vi "GenericMotionCore.vi"(5 "NumOfAxis":i32=3, 6 "MotorDisabled":refnum<vi>, 7 "Simulation":bool, 8 "error in":errorcluster, 9 "Serial Configuration":T1={"Baud Rate"=115200, "Parity"=0, "Data Bits"=8, "Stop Bits"=10, "Flow Control"=0} {"Flow Control" items=["None", "XON/XOFF", "RTS/CTS", "XON/XOFF & RTS/CTS", "DTR/DSR", "XON/XOFF & DTR/DSR"]; "Stop Bits" items=["1.0"=10, "1.5"=15, "2.0"=20]; "Data Bits" items=["7"=7, "8"=8]; "Parity" items=["None", "Odd", "Even", "Mark", "Space"]; "Baud Rate" items=["300"=300, "600"=600, "1200"=1200, "2400"=2400, "4800"=4800, "9600"=9600, "19200"=19200]}, 10 "CommPort":refnum<visa-resource-name>, 11 "ControlQueue in":refnum<queue>) -> (0 "error out":errorcluster, 3 "queue out":refnum<queue>)   [LabVIEW 2013, in "GenericMotionCore.lvlib"]
uses:
  <instrlib>/GenericMotionCore/GenericMotionCore.lvlib
  <instrlib>/GenericMotionCore/Public/Data/GenericMotion_State.ctl
  <instrlib>/GenericMotionCore/Public/Data/GenericMotion_Data.ctl
  <vilib>/Utility/error.llb/DialogType.ctl
  <instrlib>/GenericMotionCore/Public/Position_Generic.vi
panel:
  out "update_counter":i32
  in  "SoftReset":bool caption="Go"
  in  "Go_MoveRel":bool caption="Go"
  out "WaitStopBlink":i32
  out "tick_start":u32
  out "tick_stop":u32
  out "Returned_String":string
  out "refresh rate":i32
  in  "MotorDisabled":bool caption="Go"
  in  "Home":bool caption="Go"
  in  "StepWidth":dbl(ring)=0.2 items=["0.2 um"=0.0002, "0.001 mm"=0.001, "0.002 mm"=0.002, "0.005 mm "=0.005, "0.01 mm"=0.01, "0.02 mm"=0.02, "0.05 mm"=0.05, "0.1 mm"=0.1, "0.2 mm"=0.2, "1 mm"=1.0]
  in  "Z-":bool
  in  "Z+":bool
  in  "X+":bool
  in  "X-":bool
  in  "Y-":bool
  in  "Y+":bool
  in  "ClearErr":bool caption="Go"
  in  "STOP":bool caption="Go"
  in  "Quit":bool caption="Go"
  in  "SetPosition":dbl[](array[numeric])=[1.0, 1.0, 1.0] caption="Position" format="%.4f"
  in  "SetVelocity":dbl[](array[numeric])=[1.0] caption="Velocity"
  in  "SetAcceleration":dbl[](array[numeric])=[50.0] caption="Acceleration"
  in  "Go":bool
  out "Moving":bool
  out "Acceleration":dbl[](array[numeric])
  out "Velocity":dbl[](array[numeric])
  out "Position":dbl[](array[numeric])
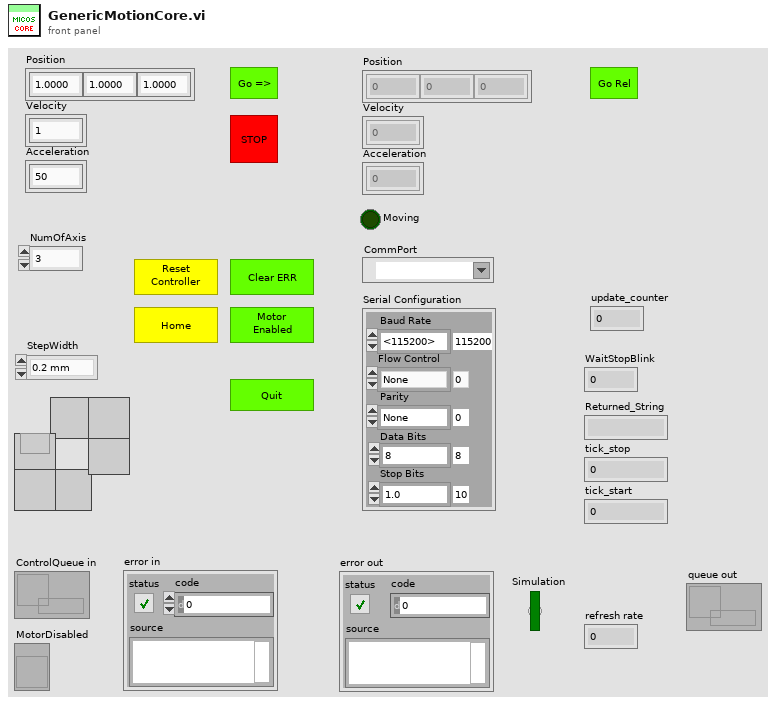
[diagram p1: front panel]
types:
  T1 = cluster{"Baud Rate":u32, "Parity":u16, "Data Bits":u16, "Stop Bits":u16, "Flow Control":u16}
  T2 = cluster{"Acceleration":dbl[], "Velocity":dbl[], "tick_move_target":u32, "Position target":dbl[], "Velocity_axial":dbl[]}
  T3 = cluster{"Position_Target":dbl[], "Velocity_axial":dbl[], "Acceleration":dbl[], "Moving":bool, "Simulation":bool, "tick_MoveTarget":u32, "NumOfAxis":i32, "Range":dbl[][]}
  T4 = cluster{"CommPort":refnum<vi>, "Serial Configuration":refnum<vi>, "SetPosition":refnum<vi>, "SetAcceleration":refnum<vi>, "SetVelocity":refnum<vi>, "StepWidth":refnum<vi>, "WaitStopReturn_Queue":refnum<queue>}
  T5 = typedef "GenericMotionCore.lvlib/GenericMotion_State.ctl" = cluster{"State":enum16{"Initialize", "SetDefaultConfig", "Close", "Quit", "Identify", "MoveAbs", "MoveAbs_all", "MoveRel", "MoveRel_all", "STOP", "Origin/Home", "WaitStop", "QueryStatus", "UpdateXPos", "UpdateAll", "SetVelocity", "SetAcceleration", "ClearErr", "LogMessage", "MotorEnable(1)", "EnableAxis", "JoyStick", "GetVelocity", "GetAcceleration", "SendCmd", "SetSoftLimits", "Beep", "_SettingReturn", "SoftReset"}, "Params.":variant}
  T6 = typedef "GenericMotionCore.lvlib/GenericMotion_Data.ctl" = cluster{"Position":dbl[], "Velocity":dbl[], "Acceleration":dbl[], "Moving":bool, "Simulation":bool, "tickcount_mov":u32, "tickcount_pos":u32, "NumOfAxis":i32, "Initialized":bool, "CommPort":refnum<visa-resource-name>, "Range":dbl[][], "Serial Configuration":cluster{"Baud Rate":u32, "Parity":u16, "Data Bits":u16, "Stop Bits":u16, "Flow Control":u16}, "MotorDisabled":refnum<vi>}
  T7 = typedef "StepWidthSelector.ctl" = dbl
  T8 = enum16{"Initialize", "SetDefaultConfig", "Close", "Quit", "Identify", "MoveAbs", "MoveAbs_all", "MoveRel", "MoveRel_all", "STOP", "Origin/Home", "WaitStop", "QueryStatus", "UpdateXPos", "UpdateAll", "SetVelocity", "SetAcceleration", "ClearErr", "LogMessage", "MotorEnable(1)", "EnableAxis", "JoyStick", "GetVelocity", "GetAcceleration", "SendCmd", "SetSoftLimits", "Beep", "_SettingReturn"}
  T9 = enum16{"Initialize", "SetDefaultConfig", "Close", "Quit", "Identify", "MoveAbs", "MoveAbs_all", "MoveRel", "MoveRel_all", "STOP", "Origin/Home", "WaitStop", "QueryStatus", "UpdateXPos", "UpdateAll", "SetVelocity", "SetAcceleration", "ClearErr", "LogMessage", "MotorEnable(1)", "EnableAxis", "JoyStick", "GetVelocity", "GetAcceleration", "SendCmd", "SetSoftLimits", "Beep", "_SettingReturn", "SoftReset"}
  T10 = typedef "DialogType.ctl" = u16
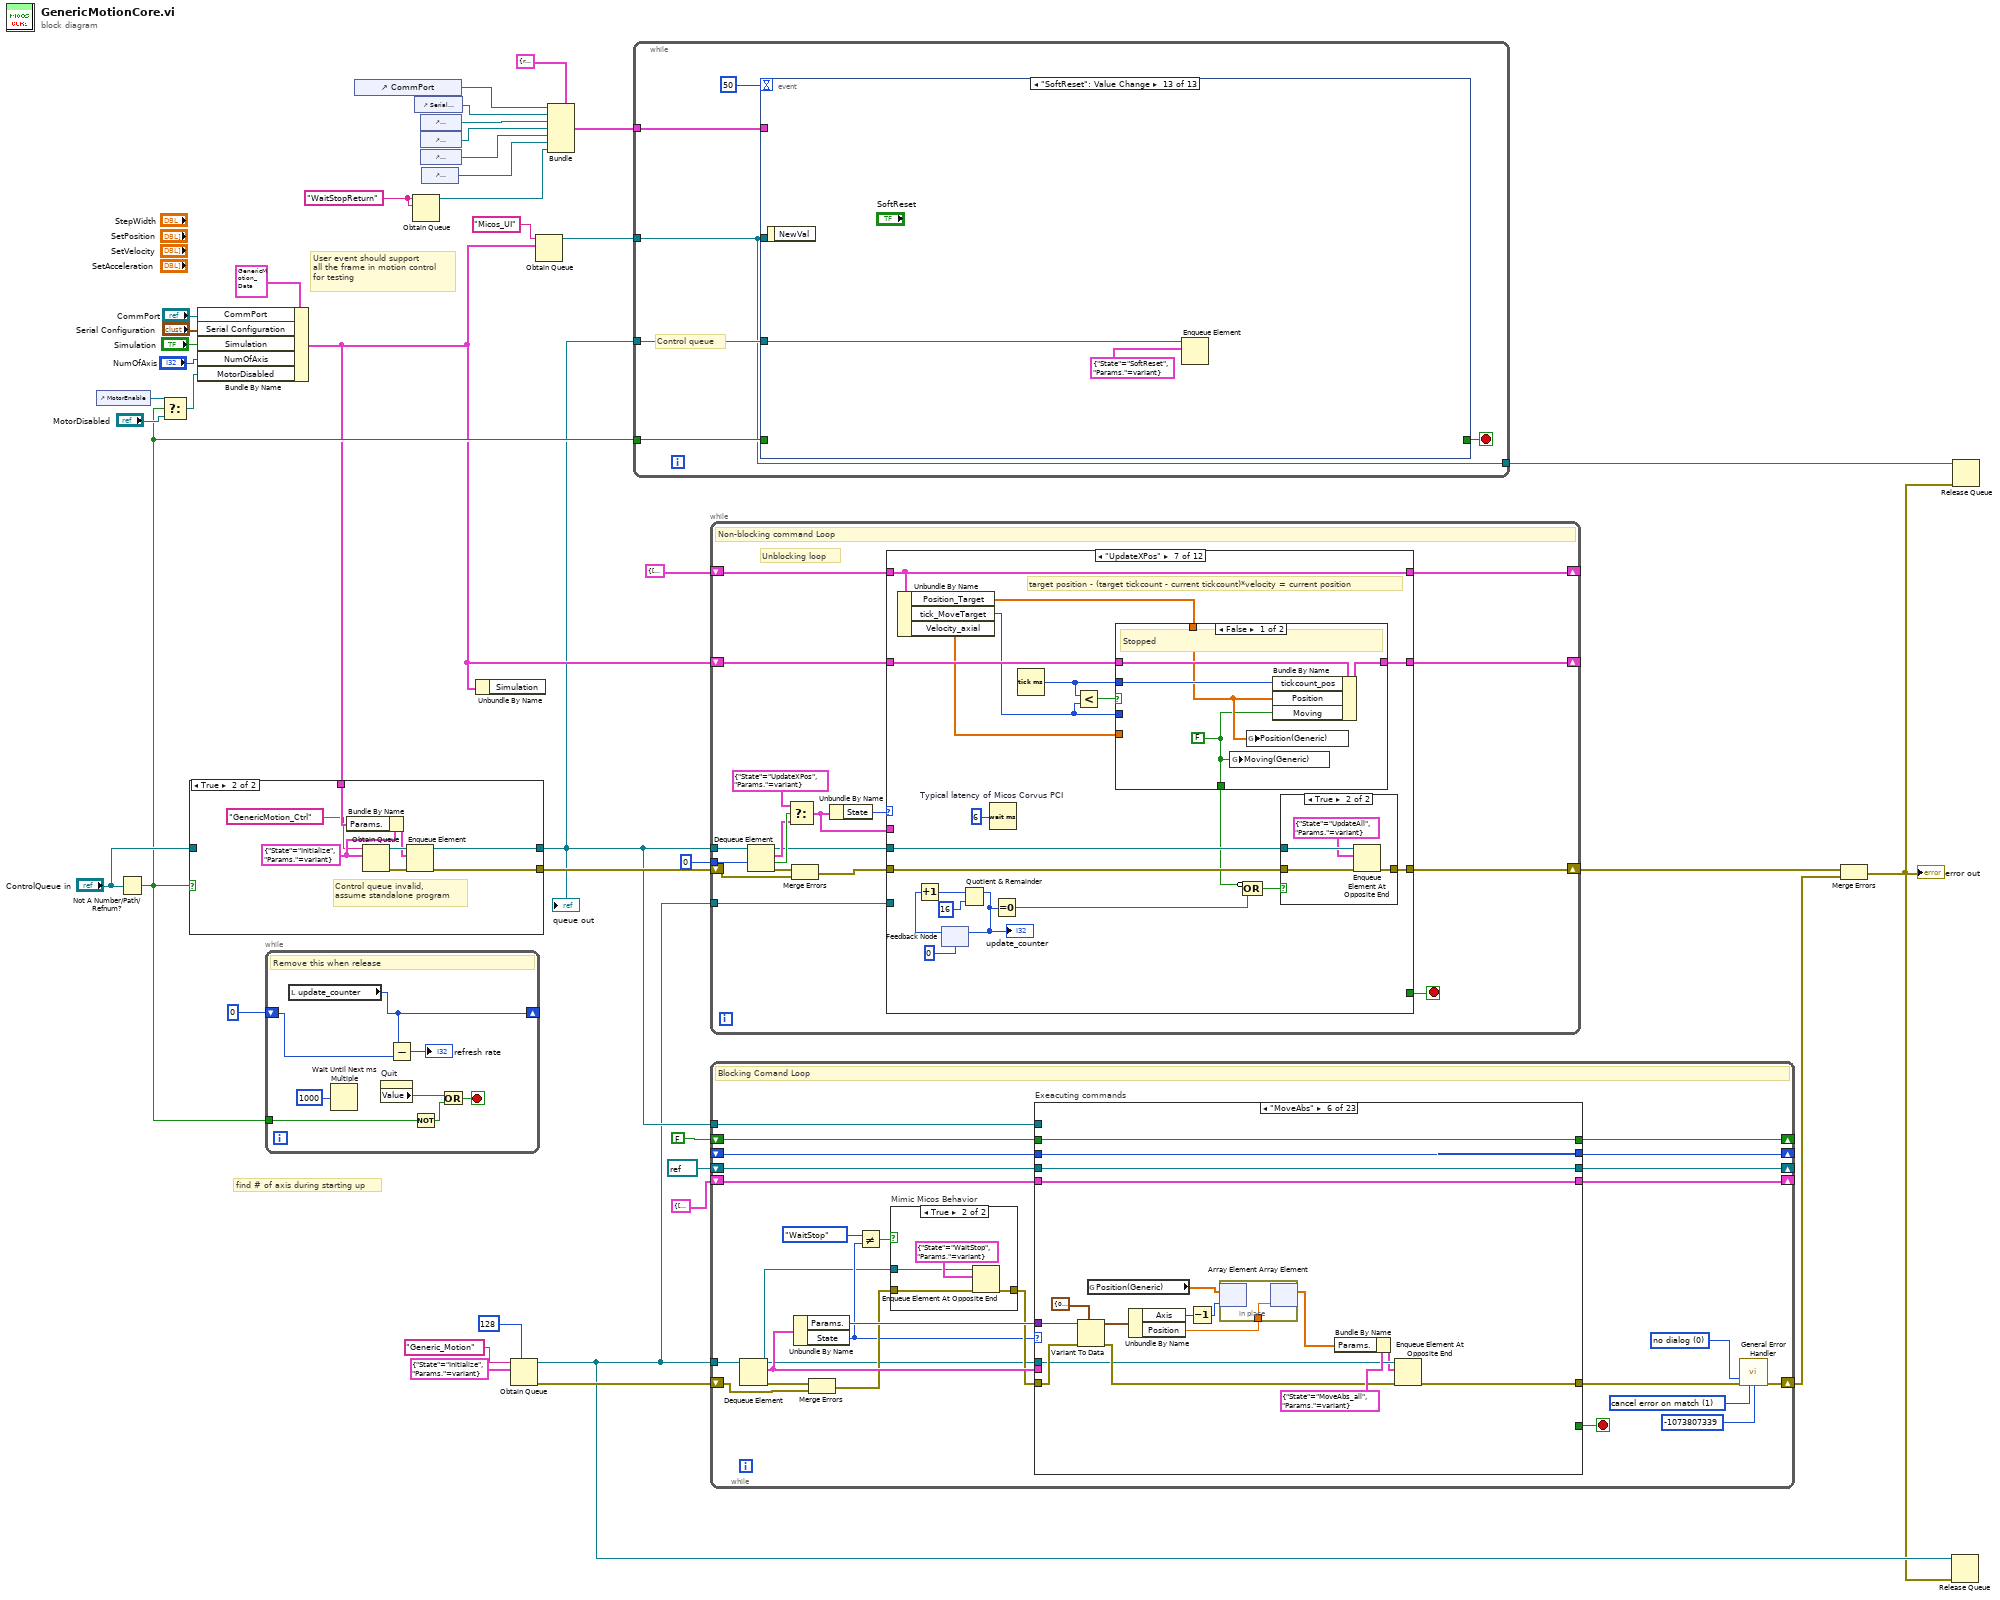
[diagram p0: block diagram]
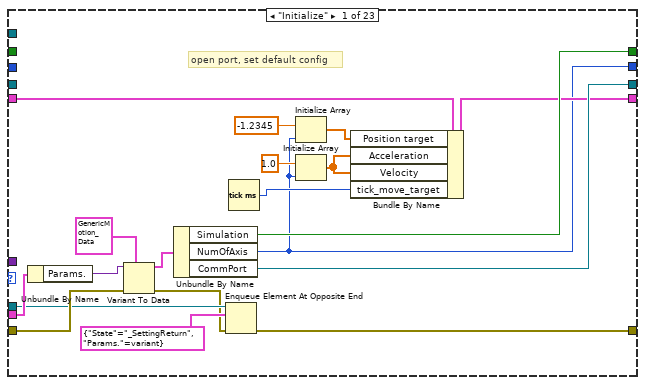
[diagram p3: hidden frame]
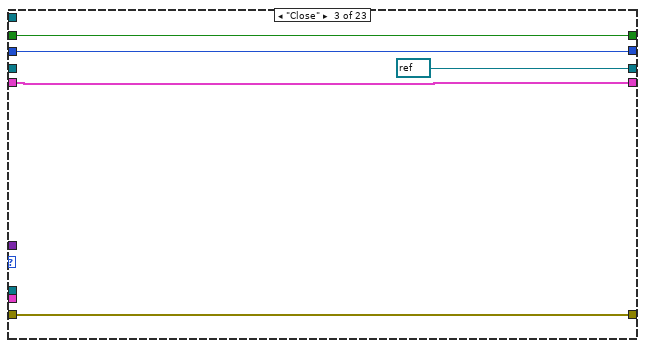
[diagram p5: hidden frame]
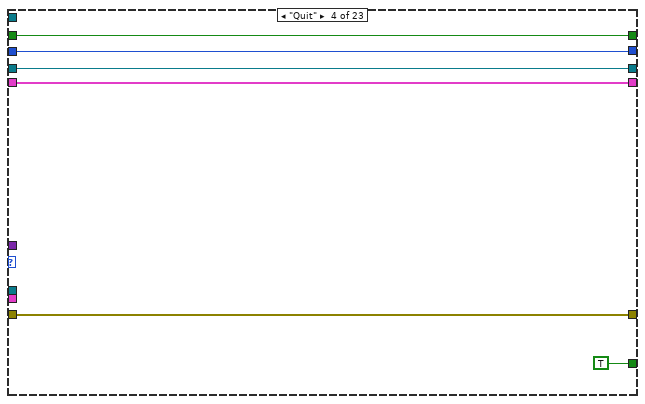
[diagram p6: hidden frame]
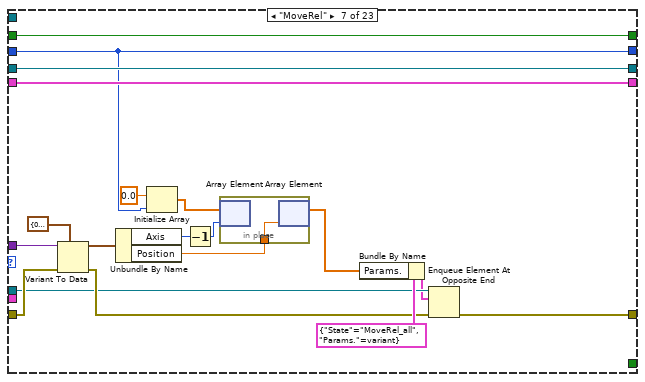
[diagram p8: hidden frame]
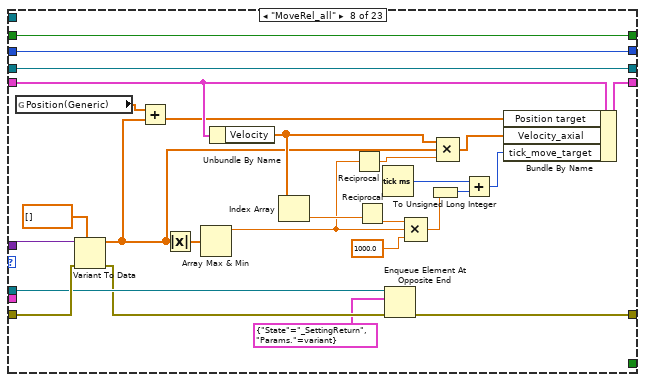
[diagram p9: hidden frame]
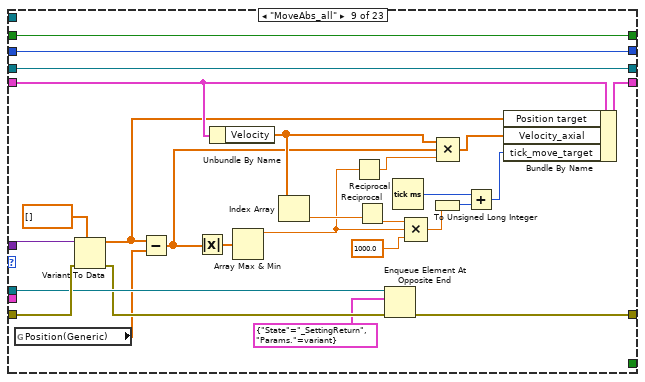
[diagram p10: hidden frame]
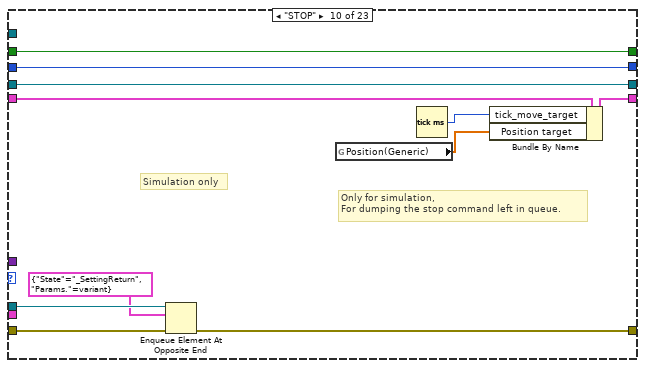
[diagram p11: hidden frame]
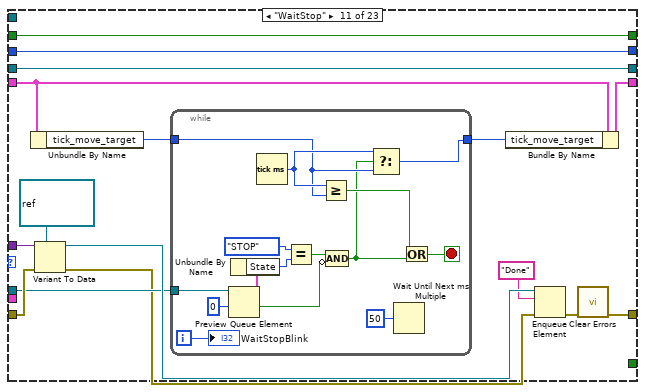
[diagram p12: hidden frame]
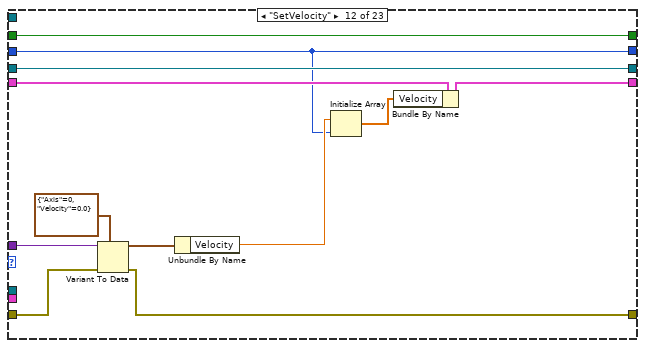
[diagram p13: hidden frame]
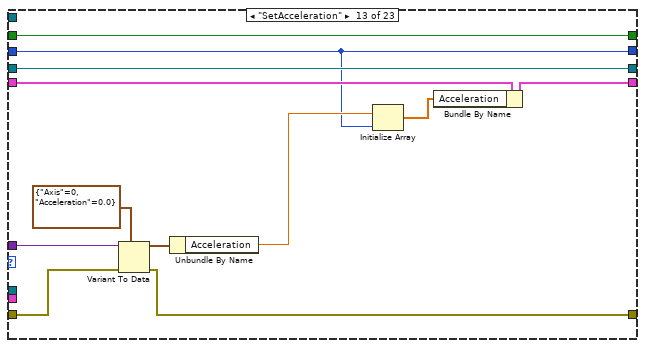
[diagram p14: hidden frame]
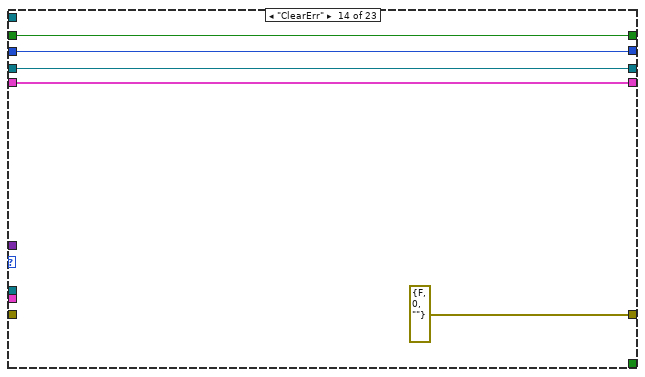
[diagram p15: hidden frame]
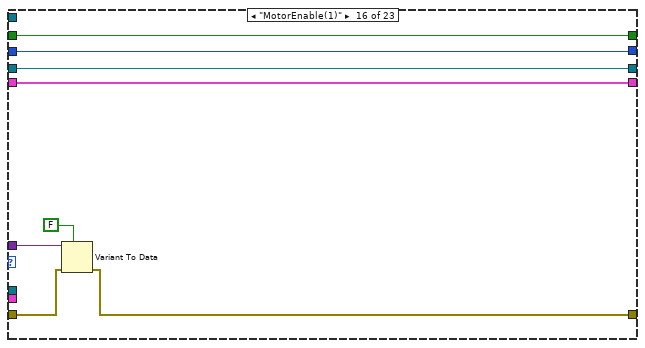
[diagram p17: hidden frame]
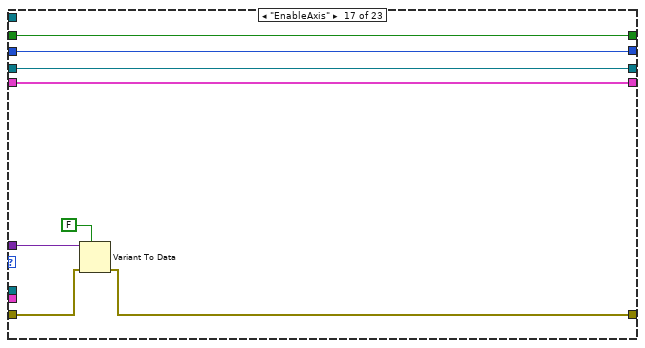
[diagram p18: hidden frame]
diagram:
  w15 = "WaitStopReturn" ("name (unnamed)")
  # "find # of axis during starting up"
  # "User event should support \nall the frame in motion control\nfor testing"
  n1 = control-ref of="MotorEnable"() -> (w22:refnum<vi>)
  n2 = Not A Number/Path/Refnum?(number/path/refnum="ControlQueue in") -> (NaN/Path/Refnum?=w17:bool)
  n3 = Select(t=w22, s=w17, f="MotorDisabled") -> (s? t:f=w20:refnum<vi>)
  n4 = Bundle By Name(cluster=T6 {"Position"=[], "Velocity"=[], "Acceleration"=[], "Moving"=FALSE, "Simulation"=FALSE, "tickcount_mov"=0, "tickcount_pos"=0, "NumOfAxis"=0, "Initialized"=FALSE, "CommPort"="", "Range"=[], "Serial Configuration"={"Baud Rate"=0, "Parity"=0, "Data Bits"=0, "Stop Bits"=0, "Flow Control"=0}, "MotorDisabled"=refnum}, "CommPort"="CommPort", "Serial Configuration"="Serial Configuration", "Simulation"="Simulation", "NumOfAxis"="NumOfAxis", "MotorDisabled"=w20) -> (w16:T6)
  n5 = case shown="True" w17 {
    tunnel: [w42 w48] -> w11
    tunnel: ["error in" w47] -> w40
    tunnel: "ControlQueue in" -> [w42 _]
    tunnel: w16 -> [_ w44]
    frame False {
    }
    frame True {
      w49 = T5 {"State"=enum."Initialize", "Params."=variant}
      # "Control queue invalid, \nassume standalone program"
      n6 = Bundle By Name(cluster=w49, "Params."=w44) -> (w45:T5)
      n7 = Obtain Queue(name (unnamed)="GenericMotion_Ctrl", element data type=w49) -> (queue out=w50:refnum<queue>, error out=w46:errorcluster)  [unwired: 3 in, 1 out]
      n8 = Enqueue Element(queue=w50, element=w45, error in (no error)=w46) -> (queue out=w48:refnum<queue>, error out=w47:errorcluster)  [unwired: 1 in, 1 out]
    }
  }
  "queue out" <- w11
  n9 = while {
    shift-right: [w51] -> _
    shift-left: 0 ("resfresh counter") -> [w58]
    tunnel: w17 -> [w53]
    stop <- w54 stop-if-true
    # "Remove this when release"
    n10 = local read "update_counter"() -> (w51:i32)
    n11 = Wait Until Next ms Multiple(millisecond multiple=u32 1000) -> ()  [unwired: 1 out]
    n12 = property on="Quit" class="Bool (strict)"() -> ("Value"=w56:bool)  [unwired: 2 in, 2 out]
    n13 = Subtract(x=w51, y=w58) -> (x-y=→"refresh rate":i32)
    n14 = Not(x=w53) -> (.not. x?=w52:bool)
    n15 = Or(x=w56, y=w52) -> (x .or. y?=w54:bool)
  }
  n16 = control-ref of="CommPort"() -> (w32:refnum<vi>)
  n17 = Obtain Queue(name (unnamed)=w15, element data type=w15) -> (queue out=w14:refnum<queue>)  [unwired: 3 in, 2 out]
  n18 = control-ref of="Serial Configuration"() -> (w33:refnum<vi>)
  n19 = control-ref of="SetPosition"() -> (w31:refnum<vi>)
  n20 = control-ref of="SetAcceleration"() -> (w30:refnum<vi>)
  n21 = control-ref of="SetVelocity"() -> (w29:refnum<vi>)
  n22 = control-ref of="StepWidth"() -> (w23:refnum<vi>)
  n23 = Unbundle By Name(w16) -> ()  [unwired: 1 out]
  n24 = Obtain Queue(max queue size (-1, unlimited)=128, name (unnamed)="Generic_Motion", element data type=T5 {"State"=enum."Initialize", "Params."=variant}) -> (queue out=w9:refnum<queue>, error out=w37:errorcluster)  [unwired: 2 in, 1 out]
  n25 = Obtain Queue(name (unnamed)="Micos_UI", element data type=w16) -> (queue out=w12:refnum<queue>)  [unwired: 3 in, 2 out]
  n26 = Bundle(cluster=T4 {"CommPort"=refnum, "Serial Configuration"=refnum, "SetPosition"=refnum, "SetAcceleration"=refnum, "SetVelocity"=refnum, "StepWidth"=refnum, "WaitStopReturn_Queue"=refnum}, "CommPort"=w32, "Serial Configuration"=w33, "SetPosition"=w31, "SetAcceleration"=w30, "SetVelocity"=w29, "StepWidth"=w23, "WaitStopReturn_Queue"=w14) -> (w28:T4)
  n27 = while {
    tunnel: w11 -> [w60]
    tunnel: w17 -> [w63]
    tunnel: w12 -> [w59]
    tunnel: w28 -> [w61]
    tunnel: [w59] -> w10
    stop <- w64 stop-if-true
    # "Control queue"
    n28 = event shown="[12] \"SoftReset\": Value Change" {
      selector: _ -> [_ _ _ _ _ _ _ _ _ _ _ _ _]
      dyn-events: _ -> [_ _ _ _ _ _ _ _ _ _ _ _ _]
      timeout: 50 -> [_ _ _ _ _ _ _ _ _ _ _ _ _]
      tunnel: [w67 _ _ _ _ _ _ _ _ _ TRUE _ _] -> w64
      tunnel: w63 -> [w80 _ _ _ _ _ _ _ _ _ _ _ _]
      tunnel: w60 -> [w79 w99 w110 w120 w124 w135 w162 w168 w170 w175 w178 w181 w183]
      tunnel: w59 -> [w72 _ _ _ _ _ _ _ _ _ _ _ _]
      tunnel: w61 -> [w71 w98 w109 _ _ _ w161 _ _ _ _ _ _]
      event Timeout {
        # "Send return queue ref"
        n29 = event-data() -> ()  [unwired: 1 in, 1 out]
        n30 = Unbundle By Name(w71) -> ("WaitStopReturn_Queue"=w66:refnum<queue>)
        n31 = Not(x=w80) -> (.not. x?=w67:bool)
        n32 = Bundle By Name(cluster=T5 {"State"=enum."QueryStatus", "Params."=variant} ("element"), "Params."=w72) -> (w77:T5)
        n33 = Enqueue Element(queue=w79, element=w77) -> (error out=w75:errorcluster)  [unwired: 2 in, 2 out]
        n34 = Dequeue Element(queue=w72, timeout in ms (-1)=1000, error in (no error)=w75) -> (element=w73:T6, timed out?=w74:bool)  [unwired: 2 out]
        n35 = case shown="False" w74 {
          tunnel: w73 -> [w88 _]
          frame False {
            n36 = Unbundle By Name(w88) -> ("Position"=→"Position":dbl[], "Velocity"=→"Velocity":dbl[], "Acceleration"=→"Acceleration":dbl[], "Moving"=→"Moving":bool)
          }
          frame True {
          }
        }
        n37 = Dequeue Element(queue=w66, timeout in ms (-1)=0) -> (queue out=w65:refnum<queue>, element=w70:string, timed out?=w69:bool)  [unwired: 1 in, 1 out]
        n38 = case "Non-blocking WaitStop in UI for testing" shown="False" w69 {
          tunnel: w70 -> [w82 _]
          frame False {
            # "Non-blocking Wait for testing"
            n39 = Tick Count (ms)() -> (millisecond timer value=→"tick_stop":u32)
            "Returned_String" <- w82
          }
          frame True {
          }
        }
        n40 = case "Release feedback queue if no UI" shown="True" w67 {
          tunnel: w65 -> [_ w81]
          frame False {
          }
          frame True {
            n41 = Release Queue(queue=w81) -> ()  [unwired: 2 in, 3 out]
          }
        }
      }
      event "Go": Value Change {
        n42 = Unbundle By Name(w98) -> ("WaitStopReturn_Queue"=w93:refnum<queue>, "SetPosition"=w97:refnum<vi>)
        n43 = event-data() -> ()  [unwired: 1 in, 1 out]
        n44 = flat-sequence {
          tunnel: w99 -> [w106]
          tunnel: w96 -> [w103]
          tunnel: [w102] -> w95
          tunnel: [w101] -> w94
          frame #0 {
            n45 = Tick Count (ms)() -> (millisecond timer value=→"tick_start":u32)
            n46 = Bundle By Name(cluster=T5 {"State"=enum."MoveAbs_all", "Params."=variant} ("element"), "Params."=w103) -> (w104:T5)
            n47 = Enqueue Element(queue=w106, element=w104) -> (queue out=w102:refnum<queue>, error out=w101:errorcluster)  [unwired: 2 in, 1 out]
          }
        }
        n48 = property class="Arr (strict)"(reference=w97) -> ("Value"=w96:dbl[])  [unwired: 1 in, 2 out]
        n49 = local write "Returned_String"("Done" ("Returned_String")) -> ()
        n50 = local write "tick_stop"(u32 0 ("tick_stop")) -> ()
        n51 = Bundle By Name(cluster=T5 {"State"=enum."WaitStop", "Params."=variant} ("element"), "Params."=w93) -> (w90:T5)
        n52 = Enqueue Element(queue=w95, element=w90, error in (no error)=w94) -> ()  [unwired: 1 in, 3 out]
      }
      event "Go_MoveRel": Value Change {
        n53 = event-data() -> ()  [unwired: 1 in, 1 out]
        n54 = Unbundle By Name(w109) -> ("SetPosition"=w108:refnum<vi>)
        n55 = flat-sequence {
          tunnel: w110 -> [w116]
          tunnel: w107 -> [w113]
          tunnel: [w112] -> _
          tunnel: [w111] -> _
          frame #0 {
            n56 = Bundle By Name(cluster=T5 {"State"=enum."MoveRel_all", "Params."=variant} ("element"), "Params."=w113) -> (w114:T5)
            n57 = Enqueue Element(queue=w116, element=w114) -> (queue out=w112:refnum<queue>, error out=w111:errorcluster)  [unwired: 2 in, 1 out]
          }
        }
        n58 = property class="Arr (strict)"(reference=w108) -> ("Value"=w107:dbl[])  [unwired: 1 in, 2 out]
      }
      event "SetPosition": Value Change {
        n59 = event-data() -> ("NewVal"=w117:dbl[])  [unwired: 1 in]
        n60 = Bundle By Name(cluster=T5 {"State"=enum."MoveAbs_all", "Params."=variant} ("element"), "Params."=w117) -> (w118:T5)
        n61 = Enqueue Element(queue=w120, element=w118) -> ()  [unwired: 2 in, 3 out]
      }
      event "SetVelocity": Value Change {
        n62 = event-data() -> ("NewVal"=w123:dbl[])  [unwired: 1 in]
        n63 = for {
          tunnel: w123 -> [w126] mode=indexing
          shift-right: [w125] -> w122
          shift-left: w124 -> [w125]
          i -> [w132]
          n64 = Increment(x=w132) -> (x+1=w130:i32)
          n65 = Bundle By Name(cluster=cluster{"Axis":i32, "Velocity":dbl} {"Axis"=0, "Velocity"=0.0}, "Velocity"=w126, "Axis"=w130) -> (w127:cluster{"Axis":i32, "Velocity":dbl})
          n66 = Bundle By Name(cluster=T5 {"State"=enum."SetVelocity", "Params."=variant} ("element"), "Params."=w127) -> (w129:T5)
          n67 = Enqueue Element(queue=w125, element=w129) -> ()  [unwired: 2 in, 3 out]
        }
        n68 = Enqueue Element(queue=w122, element=T5 {"State"=enum."GetVelocity", "Params."=variant}) -> ()  [unwired: 2 in, 3 out]
      }
      event "SetAcceleration": Value Change {
        n69 = event-data() -> ("NewVal"=w136:dbl[])  [unwired: 1 in]
        n70 = for {
          tunnel: w136 -> [w138] mode=indexing
          shift-right: [w137] -> w133
          shift-left: w135 -> [w137]
          i -> [w144]
          n71 = Increment(x=w144) -> (x+1=w142:i32)
          n72 = Bundle By Name(cluster=cluster{"Axis":i32, "Acceleration":dbl} {"Axis"=0, "Acceleration"=0.0}, "Acceleration"=w138, "Axis"=w142) -> (w139:cluster{"Axis":i32, "Acceleration":dbl})
          n73 = Bundle By Name(cluster=T5 {"State"=enum."SetAcceleration", "Params."=variant} ("element"), "Params."=w139) -> (w141:T5)
          n74 = Enqueue Element(queue=w137, element=w141) -> ()  [unwired: 2 in, 3 out]
        }
        n75 = Enqueue Element(queue=w133, element=T5 {"State"=enum."GetAcceleration", "Params."=variant}) -> ()  [unwired: 2 in, 3 out]
      }
      event "X+", "X-", "Y+", "Y-", "Z+", "Z-": Value Change {
        n76 = event-data() -> ()  [unwired: 1 in, 1 out]
        n77 = Unbundle By Name(w161) -> ("StepWidth"=w160:refnum<vi>)
        n78 = property class="Ring (strict)"(reference=w160) -> ("Value"=w152:T7)  [unwired: 1 in, 2 out]
        n79 = Build Array("X+", "X-", "Y+", "Y-", "Z+", "Z-") -> (w159:bool[])
        n80 = Search 1D Array(1D array=w159, element=TRUE) -> (index of element=w156:i32)  [unwired: 1 in]
        n81 = Index Array(array=dbl[] [1.0, -1.0, 1.0, -1.0, 1.0, -1.0], index=w156) -> (element=w155:dbl)
        n82 = Index Array(array=i32[] [1, 1, 2, 2, 3, 3], index=w156) -> (element=w151:i32)
        n83 = Multiply(x=w152, y=w155) -> (x*y=w153:T7)
        n84 = Bundle By Name(cluster=cluster{"Axis":i32, "Position":dbl} {"Axis"=0, "Position"=0.0}, "Position"=w153, "Axis"=w151) -> (w163:cluster{"Axis":i32, "Position":dbl})
        n85 = Bundle By Name(cluster=T5 {"State"=enum."MoveRel", "Params."=variant} ("element"), "Params."=w163) -> (w165:T5)
        n86 = Enqueue Element(queue=w162, element=w165) -> ()  [unwired: 2 in, 3 out]
      }
      event "STOP": Value Change {
        n87 = event-data() -> ()  [unwired: 1 in, 1 out]
        n88 = Enqueue Element(queue=w168, element=T5 {"State"=enum."STOP", "Params."=variant}) -> ()  [unwired: 2 in, 3 out]
      }
      event "Home": Value Change {
        n89 = event-data() -> ()  [unwired: 1 in, 1 out]
        n90 = Enqueue Element(queue=w170, element=T5 {"State"=enum."Origin/Home", "Params."=variant}) -> ()  [unwired: 2 in, 3 out]
      }
      event "MotorDisabled": Value Change {
        n91 = event-data() -> ()  [unwired: 1 in, 1 out]
        n92 = Not(x="MotorDisabled") -> (.not. x?=w171:bool)
        n93 = Bundle By Name(cluster=T5 {"State"=enum."MotorEnable(1)", "Params."=variant} ("element"), "Params."=w171) -> (w173:T5)
        n94 = Enqueue Element(queue=w175, element=w173) -> ()  [unwired: 2 in, 3 out]
      }
      event "Quit": Value Change {
        n95 = event-data() -> ()  [unwired: 1 in, 1 out]
        n96 = disable-structure shown="Disabled" {
          frame Disabled {
            n97 = property on="Quit" class="Bool (strict)"("Value"=FALSE ("Quit")) -> ()  [unwired: 2 in, 2 out]
          }
          frame Enabled {
          }
        }
        n98 = Enqueue Element(queue=w178, element=T5 {"State"=enum."Quit", "Params."=variant}) -> ()  [unwired: 2 in, 3 out]
      }
      event "ClearErr": Value Change {
        n99 = event-data() -> ()  [unwired: 1 in, 1 out]
        n100 = Enqueue Element(queue=w181, element=T5 {"State"=enum."ClearErr", "Params."=variant}) -> ()  [unwired: 2 in, 3 out]
      }
      event "SoftReset": Value Change {
        n101 = event-data() -> ()  [unwired: 1 in, 1 out]
        n102 = Enqueue Element(queue=w183, element=T5 {"State"=enum."SoftReset", "Params."=variant}) -> ()  [unwired: 2 in, 3 out]
      }
    }
  }
  n103 = while {
    tunnel: w11 -> [w191]
    shift-right: [w201] -> _
    shift-left: w16 -> [w200]
    tunnel: w9 -> [w198]
    shift-right: [w186] -> w4
    shift-left: w40 -> [w187]
    tunnel: 0 ("f") -> [w189]
    shift-right: [w185] -> _
    shift-left: T3 {"Position_Target"=[], "Velocity_axial"=[], "Acceleration"=[], "Moving"=FALSE, "Simulation"=FALSE, "tick_MoveTarget"=0, "NumOfAxis"=0, "Range"=[]} ("output cluster") -> [w184]
    stop <- w199 stop-if-true
    # "Unblocking loop"
    # "Non-blocking command Loop"
    n104 = Dequeue Element(queue=w191, timeout in ms (-1)=w189) -> (queue out=w192:refnum<queue>, element=w194:T5, timed out?=w196:bool, error out=w197:errorcluster)  [unwired: 1 in]
    n105 = Select(t=T5 {"State"=enum."UpdateXPos", "Params."=variant} ("element"), s=w196, f=w194) -> (s? t:f=w193:T5)
    n106 = Merge Errors(w197, w187) -> (w188:errorcluster)
    n107 = Unbundle By Name(w193) -> ("State"=w190:T9)
    n108 = case shown="\"UpdateXPos\"" w190 {
      tunnel: w193 -> [w213 w228 _ _ w289 w302 _ _ _ w380 w397 w404]
      tunnel: [w204 w225 w246 w267 w294 w298 w324 w355 w374 w383 w387 w409] -> w201
      tunnel: w200 -> [w215 w223 w246 w265 w285 w298 w322 w353 w374 w383 w398 w409]
      tunnel: [_ _ TRUE _ _ _ _ _ _ _ _ _] -> w199
      tunnel: w198 -> [w212 w229 w249 w274 w286 _ _ _ _ w382 _ w408]
      tunnel: [w214 w226 w251 w272 w287 w300 w316 w354 errorcluster {"status"=FALSE, "code"=0, "source"=""} ("error out") w379 w391 w401] -> w186
      tunnel: w188 -> [w218 w227 w247 w273 w288 w301 w323 w354 _ w381 w392 w407]
      tunnel: w192 -> [_ w221 _ _ _ _ w315 _ _ _ _ w405]
      tunnel: [w205 w220 w244 w268 w293 w296 w311 w351 w372 w375 w390 w400] -> w185
      tunnel: w184 -> [w211 w220 w244 w269 w295 w296 w311 w351 w372 w375 w393 w400]
      frame "Initialize" {
        # "cmd +(stage data)"
        # "stage data"
        n109 = Unbundle By Name(w213) -> ("Params."=w219:variant)
        n110 = Variant To Data(error in=w218, type=w215, Variant=w219) -> (data=w216:T6, error out=w217:errorcluster)
        n111 = Select(t=w215, s=w217, f=w216) -> (s? t:f=w207:T6)
        n112 = call <vilib>:"Clear Errors.vi"("error in (no error)"=w217) -> ("error out"=w214:errorcluster)  [unwired: 6 in]
        n113 = Unbundle By Name(w207) -> ("NumOfAxis"=w206:i32)
        n114 = Initialize Array(-1.2345 ("element"), w206) -> (w203:dbl[])
        n115 = global write "Position_Generic.vi" "Position(Generic)"(w203) -> ()
        n116 = Bundle By Name(cluster=w211, "Position_Target"=w203) -> (w205:T3)
        n117 = Bundle By Name(cluster=w207, "Position"=w203, "Initialized"=TRUE) -> (w204:T6)
        n118 = Bundle By Name(cluster=T5 {"State"=enum."Initialize", "Params."=variant}, "Params."=w207) -> (w210:T5)
        n119 = Enqueue Element(queue=w212, element=w210) -> ()  [unwired: 2 in, 3 out]
      }
      frame "Close" {
        n120 = Unbundle By Name(w223) -> ("Moving"=w222:bool)
        n121 = case shown="True" w222 {
          tunnel: w229 -> [w233 _]
          tunnel: w228 -> [w232 w234]
          tunnel: w227 -> [w231 w238]
          tunnel: [w230 w235] -> w226
          tunnel: w221 -> [_ w243]
          frame False {
            n122 = Enqueue Element(queue=w233, element=w232, error in (no error)=w231) -> (error out=w230:errorcluster)  [unwired: 1 in, 2 out]
          }
          frame True {
            n123 = Enqueue Element At Opposite End(queue=w243, element=w234, error in (no error)=w238) -> (queue out=w242:refnum<queue>, error out=w237:errorcluster)  [unwired: 1 in, 1 out]
            n124 = Enqueue Element At Opposite End(queue=w242, element=T5 {"State"=enum."UpdateAll", "Params."=variant}, error in (no error)=w237) -> (queue out=w241:refnum<queue>, error out=w236:errorcluster)  [unwired: 1 in, 1 out]
            n125 = Enqueue Element At Opposite End(queue=w241, element=T5 {"State"=enum."STOP", "Params."=variant}, error in (no error)=w236) -> (error out=w235:errorcluster)  [unwired: 1 in, 2 out]
          }
        }
        n126 = Bundle By Name(cluster=w223, "Initialized"=FALSE) -> (w225:T6)
      }
      frame "Quit" {
        n127 = Unbundle By Name(w246) -> ("Initialized"=w245:bool)
        n128 = case shown="False" w245 {
          tunnel: [w255 w259] -> w250
          tunnel: w249 -> [w255 w258]
          tunnel: [w254 w257] -> w248
          tunnel: w247 -> [w254 w256]
          frame False {
          }
          frame True {
            n129 = Enqueue Element(queue=w258, element=T5 {"State"=enum."Close", "Params."=variant}, error in (no error)=w256) -> (queue out=w259:refnum<queue>, error out=w257:errorcluster)  [unwired: 1 in, 1 out]
          }
        }
        n130 = Enqueue Element(queue=w250, element=T5 {"State"=enum."Quit", "Params."=variant}, error in (no error)=w248) -> (error out=w251:errorcluster)  [unwired: 1 in, 2 out]
      }
      frame "STOP" {
        # "should not dump wait for stop!!"
        # "send stop to controller, update"
        n131 = Flush Queue(queue=w274, error in (no error)=w273) -> (queue out=w270:refnum<queue>, remaining elements=w271:T5[], error out=w272:errorcluster)
        n132 = for {
          tunnel: w271 -> [w280] mode=indexing
          shift-right: [w275] -> w262
          shift-left: w270 -> [w279]
          tunnel: [w275] -> _ mode=indexing
          n133 = Unbundle By Name(w280) -> ("State"=w278:T9)
          n134 = Equal?(x=w278, y=T8."WaitStop") -> (x = y?=w276:bool)
          n135 = case shown="True" w276 {
            tunnel: w280 -> [_ w284]
            tunnel: w279 -> [w281 w283]
            tunnel: [w281 w282] -> w275
            frame False {
            }
            frame True {
              n136 = Enqueue Element At Opposite End(queue=w283, element=w284) -> (queue out=w282:refnum<queue>)  [unwired: 2 in, 2 out]
            }
          }
        }
        n137 = Unbundle By Name(w265) -> ("Position"=w264:dbl[])
        n138 = Tick Count (ms)() -> (millisecond timer value=w263:u32)
        n139 = Bundle By Name(cluster=w269, "tick_MoveTarget"=w263, "Position_Target"=w264) -> (w268:T3)
        n140 = Bundle By Name(cluster=w265, "Position"=w264, "Moving"=FALSE) -> (w267:T6)
        n141 = Enqueue Element At Opposite End "Has to be PUSH"(queue=w262, element=T5 {"State"=enum."STOP", "Params."=variant}) -> ()  [unwired: 2 in, 3 out]
      }
      frame "Origin/Home" {
        n142 = Enqueue Element(queue=w286, element=w289, error in (no error)=w288) -> (error out=w287:errorcluster)  [unwired: 1 in, 2 out]
        n143 = Unbundle By Name(w285) -> ("NumOfAxis"=w292:i32)
        n144 = Initialize Array(0.0 ("element"), w292) -> (w290:dbl[])
        n145 = Bundle By Name(cluster=w295, "Position_Target"=w290) -> (w293:T3)
        n146 = Bundle By Name(cluster=w285, "Position"=w290) -> (w294:T6)
      }
      frame "QueryStatus" {
        # "return the value to queue"
        n147 = Unbundle By Name(w302) -> ("Params."=w304:variant)
        n148 = Variant To Data(error in=w301, type=refnum<queue> refnum ("queue out"), Variant=w304) -> (data=w299:refnum<queue>, error out=w303:errorcluster)
        n149 = Enqueue Element(queue=w299, element=w298, error in (no error)=w303) -> (error out=w300:errorcluster)  [unwired: 1 in, 2 out]
      }
      frame "UpdateXPos" {
        # "target position - (target tickcount - current tickcount)*velocity = current position"
        n150 = Unbundle By Name(w311) -> ("Position_Target"=w310:dbl[], "tick_MoveTarget"=w306:u32, "Velocity_axial"=w312:dbl[])
        n151 = feedback #1(0) -> (w319:i32)
        n152 = Increment(x=w319) -> (x+1=w320:i32)
        n153 = Quotient & Remainder(x=w320, y=16) -> (x-y*floor(x/y)=w317:i32)  [unwired: 1 out]
        "update_counter" <- w317
        n154 = feedback-in #1(w317) -> ()
        n155 = Wait (ms) "Typical latency of Micos Corvus PCI"(milliseconds to wait=u32 6) -> ()  [unwired: 1 out]
        n156 = Equal To 0?(x=w317) -> (x = 0?=w314:bool)
        n157 = Tick Count (ms)() -> (millisecond timer value=w307:u32)
        n158 = Less?(x=w307, y=w306) -> (x < y?=w308:bool)
        n159 = case shown="False" w308 {
          tunnel: [w329 w340] -> w324
          tunnel: w322 -> [w328 w339]
          tunnel: w306 -> [_ w338]
          tunnel: w312 -> [_ w336]
          tunnel: w310 -> [w326 w333]
          tunnel: w307 -> [w327 w332]
          tunnel: [w325 w330] -> w305
          frame False {
            w325 = FALSE ("Moving")
            # "Stopped"
            n160 = global write "Position_Generic.vi" "Moving(Generic)"(w325) -> ()
            n161 = global write "Position_Generic.vi" "Position(Generic)"(w326) -> ()
            n162 = Bundle By Name(cluster=w328, "tickcount_pos"=w327, "Position"=w326, "Moving"=w325) -> (w329:T6)
          }
          frame True {
            w330 = TRUE ("Moving")
            # "Moving"
            n163 = Subtract(x=w338, y=w332) -> (x-y=w337:u32)
            n164 = Compound Arithmetic op=MULTIPLY(w337, w336, 0.001) -> (w334:dbl[])
            n165 = Subtract(x=w333, y=w334) -> (x-y=w331:dbl[])
            n166 = global write "Position_Generic.vi" "Position(Generic)"(w331) -> ()
            n167 = global write "Position_Generic.vi" "Moving(Generic)"(w330) -> ()
            n168 = Bundle By Name(cluster=w339, "tickcount_pos"=w332, "Position"=w331, "Moving"=w330) -> (w340:T6)
          }
        }
        n169 = Compound Arithmetic op=OR(invert w305, w314) -> (w313:bool)
        n170 = case shown="True" w313 {
          tunnel: [w341 w345] -> w316
          tunnel: w315 -> [_ w344]
          tunnel: w323 -> [w341 w342]
          frame False {
          }
          frame True {
            n171 = Enqueue Element At Opposite End(queue=w344, element=T5 {"State"=enum."UpdateAll", "Params."=variant}, error in (no error)=w342) -> (error out=w345:errorcluster)  [unwired: 1 in, 2 out]
          }
        }
      }
      frame "UpdateAll" {
        # "target position - (target tickcount - current tickcount)*velocity = current position"
        n172 = Unbundle By Name(w351) -> ("Position_Target"=w350:dbl[], "tick_MoveTarget"=w346:u32, "Velocity_axial"=w352:dbl[])
        n173 = Wait (ms) "Typical latency of Micos Corvus PCI"(milliseconds to wait=u32 6) -> ()  [unwired: 1 out]
        n174 = Tick Count (ms)() -> (millisecond timer value=w347:u32)
        n175 = Greater Or Equal?(x=w347, y=w346) -> (x >= y?=w348:bool)
        n176 = case shown="False" w348 {
          tunnel: [w366 w371] -> w355
          tunnel: w353 -> [w365 w370]
          tunnel: w346 -> [w364 _]
          tunnel: w352 -> [w362 _]
          tunnel: w350 -> [w359 w368]
          tunnel: w347 -> [w358 w369]
          frame False {
            # "Generate current position"
            n177 = Subtract(x=w364, y=w358) -> (x-y=w363:u32)
            n178 = Compound Arithmetic op=MULTIPLY(w363, w362, 0.001) -> (w360:dbl[])
            n179 = Subtract(x=w359, y=w360) -> (x-y=w357:dbl[])
            n180 = global write "Position_Generic.vi" "Position(Generic)"(w357) -> ()
            n181 = global write "Position_Generic.vi" "Moving(Generic)"(TRUE ("Moving")) -> ()
            n182 = Bundle By Name(cluster=w365, "tickcount_pos"=w358, "Position"=w357) -> (w366:T6)
          }
          frame True {
            n183 = global write "Position_Generic.vi" "Position(Generic)"(w368) -> ()
            n184 = global write "Position_Generic.vi" "Moving(Generic)"(FALSE ("Moving")) -> ()
            n185 = Bundle By Name(cluster=w370, "tickcount_pos"=w369, "Position"=w368) -> (w371:T6)
          }
        }
      }
      frame "ClearErr" {
      }
      frame "GetVelocity", "GetAcceleration" {
        # "system does not response \nafter a command is received"
        # "timeout push command back then do update?\n\npreventing blocking"
        n186 = Enqueue Element(queue=w382, element=w380, error in (no error)=w381) -> (queue out=w377:refnum<queue>, error out=w376:errorcluster)  [unwired: 1 in, 1 out]
        n187 = Enqueue Element(queue=w377, element=T5 {"State"=enum."_SettingReturn", "Params."=variant}, error in (no error)=w376) -> (error out=w379:errorcluster)  [unwired: 1 in, 2 out]
      }
      frame "_SettingReturn" {
        n188 = Unbundle By Name(w397) -> ("Params."=w396:variant)
        n189 = Variant To Data(error in=w392, type=T2 {"Acceleration"=[], "Velocity"=[], "tick_move_target"=0, "Position target"=[], "Velocity_axial"=[]}, Variant=w396) -> (data=w394:T2, error out=w391:errorcluster)
        n190 = Unbundle By Name(w394) -> ("Position target"=w389:dbl[], "Velocity_axial"=w388:dbl[], "tick_move_target"=w384:u32, "Velocity"=w386:dbl[], "Acceleration"=w385:dbl[])
        n191 = Bundle By Name(cluster=w393, "Position_Target"=w389, "Velocity_axial"=w388, "tick_MoveTarget"=w384) -> (w390:T3)
        n192 = Bundle By Name(cluster=w398, "Velocity"=w386, "Acceleration"=w385) -> (w387:T6)
      }
      frame Default {
        # "system does not response \nafter a command is received"
        # "timeout push command back then do update?\n\npreventing blocking"
        n193 = Enqueue Element(queue=w408, element=w404, timeout in ms (-1)=50, error in (no error)=w407) -> (timed out?=w402:bool, error out=w403:errorcluster)  [unwired: 1 out]
        n194 = case shown="True" w402 {
          tunnel: w405 -> [_ w422]
          tunnel: w404 -> [_ w421]
          tunnel: w403 -> [w411 w420]
          tunnel: [w411 w417] -> w401
          tunnel: [_ w412] -> w399
          frame False {
          }
          frame True {
            w415 = 50 ("timeout in ms (-1)")
            n195 = Enqueue Element At Opposite End(queue=w422, element=w421, timeout in ms (-1)=w415, error in (no error)=w420) -> (queue out=w419:refnum<queue>, timed out?=w413:bool, error out=w416:errorcluster)
            n196 = Enqueue Element At Opposite End(queue=w419, element=T5 {"State"=enum."UpdateXPos", "Params."=variant}, timeout in ms (-1)=w415, error in (no error)=w416) -> (timed out?=w414:bool, error out=w417:errorcluster)  [unwired: 1 out]
            n197 = Or(x=w413, y=w414) -> (x .or. y?=w412:bool)
          }
        }
        n198 = case shown="True" w399 {
          frame False {
          }
          frame True {
            n199 = One Button Dialog(message="queue full,time out,missing comand") -> ()  [unwired: 1 in, 1 out]
          }
        }
      }
    }
  }
  n200 = while {
    tunnel: w9 -> [w439]
    shift-right: [w436] -> w1
    shift-left: w37 -> [w437]
    shift-right: [w438] -> _
    shift-left: refnum<visa-resource-name> refnum ("CommPort") -> [w440]
    shift-right: [w446] -> _
    shift-left: _ -> [w445]
    shift-right: [w442] -> _
    shift-left: FALSE -> [w443]
    tunnel: w11 -> [w435]
    shift-right: [w434] -> _
    shift-left: T2 {"Acceleration"=[], "Velocity"=[], "tick_move_target"=0, "Position target"=[], "Velocity_axial"=[]} -> [w433]
    stop <- w448 stop-if-true
    w430 = T10 0 items=["no dialog", "OK message", "continue or stop message", "OK message + warnings", "continue/stop + warnings"] ("type of dialog (OK msg:1)")
    w431 = 1 items=["no exception", "cancel error on match", "set error on match"] ("[exception action] (none:0)")
    # "Blocking Comand Loop"
    n201 = Dequeue Element(queue=w439) -> (queue out=w423:refnum<queue>, element=w441:T5, error out=w447:errorcluster)  [unwired: 2 in, 1 out]
    n202 = Unbundle By Name(w441) -> ("Params."=w444:variant, "State"=w425:T9)
    n203 = Merge Errors(w447, w437) -> (w427:errorcluster)
    n204 = Not Equal?(x=T8."WaitStop", y=w425) -> (x != y?=w426:bool)
    n205 = case "Mimic Micos Behavior" shown="True" w426 {
      tunnel: w427 -> [w449 w452]
      tunnel: [w449 w451] -> w428
      tunnel: w423 -> [_ w450]
      frame False {
      }
      frame True {
        n206 = Enqueue Element At Opposite End(queue=w450, element=T5 {"State"=enum."WaitStop", "Params."=variant}, error in (no error)=w452) -> (error out=w451:errorcluster)  [unwired: 1 in, 2 out]
      }
    }
    n207 = case "Exeacuting commands" shown="\"MoveAbs\"" w425 {
      tunnel: w441 -> [w472 _ _ _ _ _ _ _ _ _ _ _ _ _ _ _ _ _ _ _ _ _ w715]
      tunnel: [_ _ _ TRUE _ _ _ _ _ _ _ _ _ _ _ _ _ _ _ _ _ _ _] -> w448
      tunnel: [w457 w476 w482 w487 w491 w502 w523 w544 w571 w590 w600 w637 w649 errorcluster {"status"=FALSE, "code"=0, "source"=""} ("error out") w662 w668 w677 w683 w687 w692 w695 w710 w718] -> w429
      tunnel: w428 -> [w470 w476 w482 w487 w491 w508 w528 w554 w581 w591 w601 w638 w650 _ w662 w669 w674 w683 w687 w692 w694 w710 w718]
      tunnel: [w467 w475 refnum<visa-resource-name> refnum ("CommPort") w486 w490 w510 w530 w558 w585 w597 w611 w640 w652 w656 w661 w665 w672 w682 w686 w691 w702 w709 w719] -> w438
      tunnel: w440 -> [_ w475 _ w486 w490 w510 w530 w558 w585 w597 w611 w640 w652 w656 w661 w665 w672 w682 w686 w691 w702 w709 w719]
      tunnel: w423 -> [w460 _ _ _ _ w501 w522 w546 w573 w593 w599 _ _ _ _ _ _ _ _ _ _ _ _]
      tunnel: [w454 w477 w480 w485 w493 w505 w514 w559 w586 w596 w613 w629 w641 w655 w660 w666 w673 w681 w685 w690 w701 w704 w717] -> w446
      tunnel: w445 -> [_ w477 w480 w485 w493 w505 w514 w559 w586 w596 w613 w629 w641 w655 w660 w666 w673 w681 w685 w690 w701 w704 w717]
      tunnel: w444 -> [_ _ _ _ _ w509 w529 w556 w583 _ w610 w639 w651 _ _ w667 w675 _ _ _ _ _ _]
      tunnel: w443 -> [_ w474 w479 w484 w492 w511 w531 w557 w584 w595 w612 w636 w648 w654 w659 w670 w678 w680 w688 w693 w700 w708 w716]
      tunnel: [w466 w474 w479 w484 w492 w511 w531 w557 w584 w595 w612 w636 w648 w654 w659 w670 w678 w680 w688 w693 w700 w708 w716] -> w442
      tunnel: w435 -> [_ _ _ _ _ _ _ _ _ _ _ _ _ _ _ _ _ _ _ _ w699 _ _]
      tunnel: [w464 w473 w478 w483 w489 w506 w526 w552 w579 w589 w603 w633 w645 w653 w658 w663 w671 w679 w684 w689 w696 w706 w711] -> w434
      tunnel: w433 -> [w465 w473 w478 w483 w489 w506 w526 w553 w580 w594 w605 w634 w646 w653 w658 w663 w671 w679 w684 w689 w696 w707 w711]
      frame "Initialize" {
        # "open port, set default config"
        n208 = Unbundle By Name(w472) -> ("Params."=w471:variant)
        n209 = Variant To Data(error in=w470, type=T6 {"Position"=[], "Velocity"=[], "Acceleration"=[], "Moving"=FALSE, "Simulation"=FALSE, "tickcount_mov"=0, "tickcount_pos"=0, "NumOfAxis"=0, "Initialized"=FALSE, "CommPort"="", "Range"=[], "Serial Configuration"={"Baud Rate"=0, "Parity"=0, "Data Bits"=0, "Stop Bits"=0, "Flow Control"=0}, "MotorDisabled"=refnum}, Variant=w471) -> (data=w468:T6, error out=w458:errorcluster)
        n210 = Unbundle By Name(w468) -> ("Simulation"=w466:bool, "NumOfAxis"=w454:i32, "CommPort"=w467:refnum<visa-resource-name>)
        n211 = Enqueue Element At Opposite End(queue=w460, element=T5 {"State"=enum."_SettingReturn", "Params."=variant}, error in (no error)=w458) -> (error out=w457:errorcluster)  [unwired: 1 in, 2 out]
        n212 = Tick Count (ms)() -> (millisecond timer value=w461:u32)
        n213 = Initialize Array(-1.2345 ("element"), w454) -> (w455:dbl[])
        n214 = Initialize Array(1.0 ("element"), w454) -> (w462:dbl[])
        n215 = Bundle By Name(cluster=w465, "Position target"=w455, "Acceleration"=w462, "Velocity"=w462, "tick_move_target"=w461) -> (w464:T2)
      }
      frame "SetDefaultConfig" {
      }
      frame "Close" {
      }
      frame "Quit" {
      }
      frame "Identify" {
      }
      frame "MoveAbs" {
        n216 = Variant To Data(error in=w508, type=cluster{"Axis":i32, "Position":dbl} {"Axis"=0, "Position"=0.0}, Variant=w509) -> (data=w499:cluster{"Axis":i32, "Position":dbl}, error out=w503:errorcluster)
        n217 = global read "Position_Generic.vi" "Position(Generic)"() -> (w498:dbl[])
        n218 = Unbundle By Name(w499) -> ("Axis"=w497:i32, "Position"=w495:dbl)
        n219 = Decrement(x=w497) -> (x-1=w496:i32)
        n220 = in-place {
          in-place-border: w495 -> [w512]
          n221 = in-place-array #2(w498, w496) -> ()  [unwired: 1 out]
          n222 = in-place-array #2(w512) -> (w494:dbl[])  [unwired: 1 out]
        }
        n223 = Bundle By Name(cluster=T5 {"State"=enum."MoveAbs_all", "Params."=variant} ("element"), "Params."=w494) -> (w500:T5)
        n224 = Enqueue Element At Opposite End(queue=w501, element=w500, error in (no error)=w503) -> (error out=w502:errorcluster)  [unwired: 1 in, 2 out]
      }
      frame "MoveRel" {
        n225 = Variant To Data(error in=w528, type=cluster{"Axis":i32, "Position":dbl} {"Axis"=0, "Position"=0.0}, Variant=w529) -> (data=w520:cluster{"Axis":i32, "Position":dbl}, error out=w524:errorcluster)
        n226 = Unbundle By Name(w520) -> ("Axis"=w519:i32, "Position"=w517:dbl)
        n227 = Initialize Array(0.0 ("element"), w514) -> (w513:dbl[])
        n228 = Decrement(x=w519) -> (x-1=w518:i32)
        n229 = in-place {
          in-place-border: w517 -> [w532]
          n230 = in-place-array #3(w513, w518) -> ()  [unwired: 1 out]
          n231 = in-place-array #3(w532) -> (w516:dbl[])  [unwired: 1 out]
        }
        n232 = Bundle By Name(cluster=T5 {"State"=enum."MoveRel_all", "Params."=variant} ("element"), "Params."=w516) -> (w521:T5)
        n233 = Enqueue Element At Opposite End(queue=w522, element=w521, error in (no error)=w524) -> (error out=w523:errorcluster)  [unwired: 1 in, 2 out]
      }
      frame "MoveRel_all" {
        n234 = global read "Position_Generic.vi" "Position(Generic)"() -> (w533:dbl[])
        n235 = Variant To Data(error in=w554, type=dbl[] [] ("Position"), Variant=w556) -> (data=w535:dbl[], error out=w545:errorcluster)
        n236 = Add(x=w533, y=w535) -> (x+y=w534:dbl[])
        n237 = Absolute Value(x=w535) -> (abs(x)=w537:dbl[])
        n238 = Array Max & Min(array=w537) -> (max value=w536:dbl)  [unwired: 3 out]
        n239 = Unbundle By Name(w553) -> ("Velocity"=w540:dbl[])
        n240 = Index Array(array=w540) -> (element=w539:dbl)  [unwired: 1 in]
        n241 = Reciprocal(x=w536) -> (1/x=w550:dbl)
        n242 = Reciprocal(x=w539) -> (1/x=w538:dbl)
        n243 = Tick Count (ms)() -> (millisecond timer value=w547:u32)
        n244 = Enqueue Element At Opposite End(queue=w546, element=T5 {"State"=enum."_SettingReturn", "Params."=variant}, error in (no error)=w545) -> (error out=w544:errorcluster)  [unwired: 1 in, 2 out]
        n245 = Compound Arithmetic op=MULTIPLY(w538, w536, 1000.0 ("value")) -> (w548:dbl)
        n246 = To Unsigned Long Integer(number=w548) -> (unsigned 32bit integer=w542:u32)
        n247 = Compound Arithmetic op=MULTIPLY(w540, w535, w550) -> (w551:dbl[])
        n248 = Add(x=w547, y=w542) -> (x+y=w549:u32)
        n249 = Bundle By Name(cluster=w553, "Position target"=w534, "Velocity_axial"=w551, "tick_move_target"=w549) -> (w552:T2)
      }
      frame "MoveAbs_all" {
        n250 = global read "Position_Generic.vi" "Position(Generic)"() -> (w562:dbl[])
        n251 = Variant To Data(error in=w581, type=dbl[] [] ("Position"), Variant=w583) -> (data=w561:dbl[], error out=w572:errorcluster)
        n252 = Subtract(x=w561, y=w562) -> (x-y=w560:dbl[])
        n253 = Absolute Value(x=w560) -> (abs(x)=w564:dbl[])
        n254 = Unbundle By Name(w580) -> ("Velocity"=w567:dbl[])
        n255 = Array Max & Min(array=w564) -> (max value=w563:dbl)  [unwired: 3 out]
        n256 = Index Array(array=w567) -> (element=w566:dbl)  [unwired: 1 in]
        n257 = Reciprocal(x=w563) -> (1/x=w577:dbl)
        n258 = Reciprocal(x=w566) -> (1/x=w565:dbl)
        n259 = Enqueue Element At Opposite End(queue=w573, element=T5 {"State"=enum."_SettingReturn", "Params."=variant}, error in (no error)=w572) -> (error out=w571:errorcluster)  [unwired: 1 in, 2 out]
        n260 = Tick Count (ms)() -> (millisecond timer value=w574:u32)
        n261 = Compound Arithmetic op=MULTIPLY(w565, w563, 1000.0 ("value")) -> (w575:dbl)
        n262 = To Unsigned Long Integer(number=w575) -> (unsigned 32bit integer=w569:u32)
        n263 = Compound Arithmetic op=MULTIPLY(w567, w560, w577) -> (w578:dbl[])
        n264 = Add(x=w574, y=w569) -> (x+y=w576:u32)
        n265 = Bundle By Name(cluster=w580, "Position target"=w561, "Velocity_axial"=w578, "tick_move_target"=w576) -> (w579:T2)
      }
      frame "STOP" {
        # "Simulation only"
        # "Only for simulation, \nFor dumping the stop command left in queue."
        n266 = Enqueue Element At Opposite End(queue=w593, element=T5 {"State"=enum."_SettingReturn", "Params."=variant}, error in (no error)=w591) -> (error out=w590:errorcluster)  [unwired: 1 in, 2 out]
        n267 = global read "Position_Generic.vi" "Position(Generic)"() -> (w587:dbl[])
        n268 = Tick Count (ms)() -> (millisecond timer value=w588:u32)
        n269 = Bundle By Name(cluster=w594, "tick_move_target"=w588, "Position target"=w587) -> (w589:T2)
      }
      frame "WaitStop" {
        n270 = Unbundle By Name(w605) -> ("tick_move_target"=w604:u32)
        n271 = Variant To Data(error in=w601, type=refnum<queue> refnum ("Feedback"), Variant=w610) -> (data=w608:refnum<queue>, error out=w598:errorcluster)
        n272 = while {
          tunnel: w599 -> [w614]
          tunnel: w604 -> [w626]
          tunnel: [w619] -> w602
          i -> [w618]
          stop <- w622 stop-if-true
          n273 = Preview Queue Element(queue=w614, timeout in ms (-1)=0) -> (element=w625:T5, timed out?=w615:bool)  [unwired: 1 in, 2 out]
          n274 = Unbundle By Name(w625) -> ("State"=w624:T9)
          n275 = Tick Count (ms)() -> (millisecond timer value=w627:u32)
          n276 = Equal?(x=T8."STOP" ("State"), y=w624) -> (x = y?=w620:bool)
          n277 = Greater Or Equal?(x=w627, y=w626) -> (x >= y?=w621:bool)
          n278 = Compound Arithmetic op=AND(w620, invert w615) -> (w616:bool)
          n279 = Select(t=w627, s=w616, f=w626) -> (s? t:f=w619:u32)
          n280 = Wait Until Next ms Multiple(millisecond multiple=u32 50) -> ()  [unwired: 1 out]
          n281 = Or(x=w621, y=w616) -> (x .or. y?=w622:bool)
          "WaitStopBlink" <- w618
        }
        n282 = Bundle By Name(cluster=w605, "tick_move_target"=w602) -> (w603:T2)
        n283 = Enqueue Element(queue=w608, element="Done", error in (no error)=w598) -> (error out=w606:errorcluster)  [unwired: 1 in, 2 out]
        n284 = call <vilib>:"Clear Errors.vi"("error in (no error)"=w606) -> ("error out"=w600:errorcluster)  [unwired: 6 in]
      }
      frame "SetVelocity" {
        n285 = Variant To Data(error in=w638, type=cluster{"Axis":i32, "Velocity":dbl} {"Axis"=0, "Velocity"=0.0}, Variant=w639) -> (data=w632:cluster{"Axis":i32, "Velocity":dbl}, error out=w637:errorcluster)
        n286 = Unbundle By Name(w632) -> ("Velocity"=w630:dbl)
        n287 = Initialize Array(w630, w629) -> (w631:dbl[])
        n288 = Bundle By Name(cluster=w634, "Velocity"=w631) -> (w633:T2)
      }
      frame "SetAcceleration" {
        n289 = Variant To Data(error in=w650, type=cluster{"Axis":i32, "Acceleration":dbl} {"Axis"=0, "Acceleration"=0.0}, Variant=w651) -> (data=w644:cluster{"Axis":i32, "Acceleration":dbl}, error out=w649:errorcluster)
        n290 = Unbundle By Name(w644) -> ("Acceleration"=w642:dbl)
        n291 = Initialize Array(w642, w641) -> (w643:dbl[])
        n292 = Bundle By Name(cluster=w646, "Acceleration"=w643) -> (w645:T2)
      }
      frame "ClearErr" {
      }
      frame "LogMessage" {
      }
      frame "MotorEnable(1)" {
        n293 = Variant To Data(error in=w669, type=FALSE ("On/Off"), Variant=w667) -> (error out=w668:errorcluster)  [unwired: 1 out]
      }
      frame "EnableAxis" {
        n294 = Variant To Data(error in=w674, type=FALSE ("On/Off"), Variant=w675) -> (error out=w677:errorcluster)  [unwired: 1 out]
      }
      frame "JoyStick" {
      }
      frame "GetVelocity" {
        # "Send SettingReturn is taken cared in calling loop."
      }
      frame "GetAcceleration" {
        # "Send SettingReturn is taken cared in calling loop."
      }
      frame "_SettingReturn" {
        n295 = Bundle By Name(cluster=T5 {"State"=enum."_SettingReturn", "Params."=variant} ("element"), "Params."=w696) -> (w697:T5)
        n296 = Enqueue Element(queue=w699, element=w697, error in (no error)=w694) -> (error out=w695:errorcluster)  [unwired: 1 in, 2 out]
      }
      frame "Origin/Home" {
        n297 = Initialize Array(0.0 ("element"), w704) -> (w703:dbl[])
        n298 = Bundle By Name(cluster=w707, "Position target"=w703) -> (w706:T2)
      }
      frame Default {
        n299 = Unbundle By Name(w715) -> ("State"=w713:T9)
        n300 = Format Into String(format string="\nUnsupported command:%d,\nDefault frame", w713) -> (resulting string=w714:string)  [unwired: 2 in, 1 out]
        n301 = One Button Dialog(message=w714) -> ()  [unwired: 1 in, 1 out]
      }
    }
    n302 = call <vilib>:"General Error Handler.vi"("type of dialog (OK msg:1)"=w430, "error in (no error)"=w429, "[exception action] (none:0)"=w431, "[exception code]"=-1073807339) -> ("error out"=w436:errorcluster)  [unwired: 7 in, 4 out]
  }
  n303 = Merge Errors(w4, w1) -> (w8:errorcluster)
  "error out" <- w8
  n304 = Release Queue(queue=w9, error in (no error)=w8) -> ()  [unwired: 1 in, 3 out]
  n305 = Release Queue(queue=w10, error in (no error)=w8) -> ()  [unwired: 1 in, 3 out]
